vi "Check Map Modified.vi"(11 "Map Model in":refnum<class "Map Model.lvclass">) -> (2 "Modified":bool, 3 "Map Model out":refnum<class "Map Model.lvclass">)   [LabVIEW 2020, in "Map Model.lvlib" / "Map Model.lvclass"]
uses:
  Map Model.lvclass
  Map Model.lvclass/Map Model.ctl
panel:
  # "NOTICE -- YOU MUST LEAVE THIS NOTICE IN PLACE.\n\nCopyright (c) 2017, LIANG LIU Shawn.Liu.cn@gmail.com\nAll rights reserved.\n\nRedistribution and use in source and binary forms, with or without modification, are permitted provided that the following conditions are met:\n-Redistributions of source code must retain the above copyright notice, this list of conditions and the following disclaimer.\n-Redistributions in binary form must reproduce the above copyright notice, this list of conditions and the following disclaimer in the documentation and/or other materials provided with the distribution.\n-Neither the name of the eLp nor the names of its contributors may be used to endorse or promote products derived from this software without specific prior written permission.\n\nTHIS SOFTWARE IS PROVIDED BY THE COPYRIGHT HOLDERS AND CONTRIBUTORS \"AS IS\" AND ANY EXPRESS OR IMPLIED WARRANTIES, INCLUDING, BUT NOT LIMITED TO, THE IMPLIED WARRANTIES OF MERCHANTABILITY AND FITNESS FOR A PARTICULAR PURPOSE ARE DISCLAIMED. IN NO EVENT SHALL THE COPYRIGHT HOLDER OR CONTRIBUTORS BE LIABLE FOR ANY DIRECT, INDIRECT, INCIDENTAL, SPECIAL, EXEMPLARY, OR CONSEQUENTIAL DAMAGES (INCLUDING, BUT NOT LIMITED TO, PROCUREMENT OF SUBSTITUTE GOODS OR SERVICES; LOSS OF USE, DATA, OR PROFITS; OR BUSINESS INTERRUPTION) HOWEVER CAUSED AND ON ANY THEORY OF LIABILITY, WHETHER IN CONTRACT, STRICT LIABILITY, OR TORT (INCLUDING NEGLIGENCE OR OTHERWISE) ARISING IN ANY WAY OUT OF THE USE OF THIS SOFTWARE, EVEN IF ADVISED OF THE POSSIBILITY OF SUCH DAMAGE."
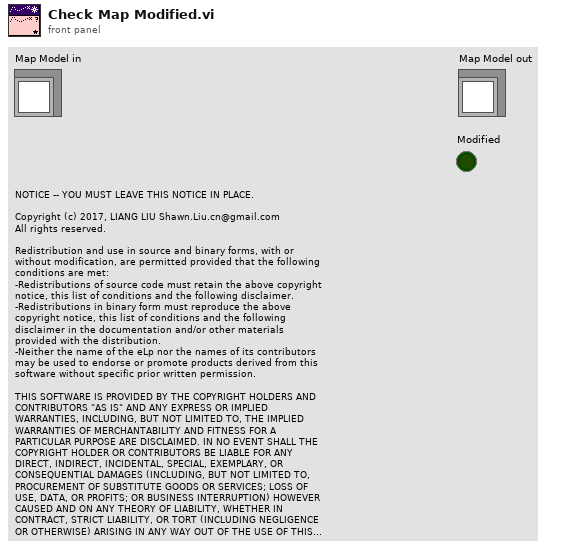
[diagram p1: front panel]
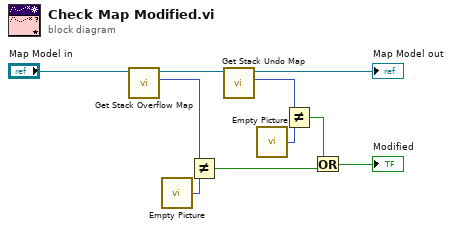
[diagram p0: block diagram]
diagram:
  n1 = call "Get Stack Overflow Map.vi"("Map Model in"="Map Model in") -> ("Stack Overflow Map"=w3:picture, "Map Model out"=w7:refnum<class "Map Model.lvclass">)  [unwired: 9 in]
  n2 = call "Empty Picture"() -> ("empty picture"=w4:picture)
  n3 = Not Equal?(x=w3, y=w4) -> (x != y?=w1:bool)
  n4 = call "Get Stack Undo Map.vi"("Map Model in"=w7) -> ("Stack Undo Map"=w6:picture, "Map Model out"=→"Map Model out":refnum<class "Map Model.lvclass">)  [unwired: 9 in]
  n5 = call "Empty Picture"() -> ("empty picture"=w5:picture)
  n6 = Not Equal?(x=w6, y=w5) -> (x != y?=w2:bool)
  n7 = Or(x=w2, y=w1) -> (x .or. y?=→"Modified":bool)
